vi "Reset VFD.vi"(6 "Direction":T1=2 items=["Reverse"=0, "Forward"=2], 8 "error In":errorcluster) -> (0 "error out":errorcluster)   [LabVIEW 2026, in "VFD Library.lvlib"]
uses:
  VFD Library.lvlib
  Action/Direction Selection.ctl
  Private/State Selection FGV.ctl
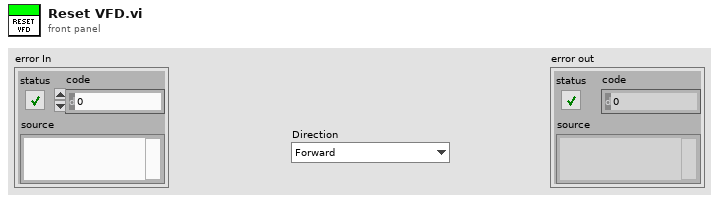
[diagram p1: front panel]
types:
  T1 = typedef "VFD Library.lvlib/Direction Selection.ctl" = u16
  T2 = typedef "State Selection FGV.ctl" = enum16{"Initilize", "Write Reg", "Write Multiple Reg", "Read Reg", "Write Coil", "Read Coil", "Reset", "Close"}
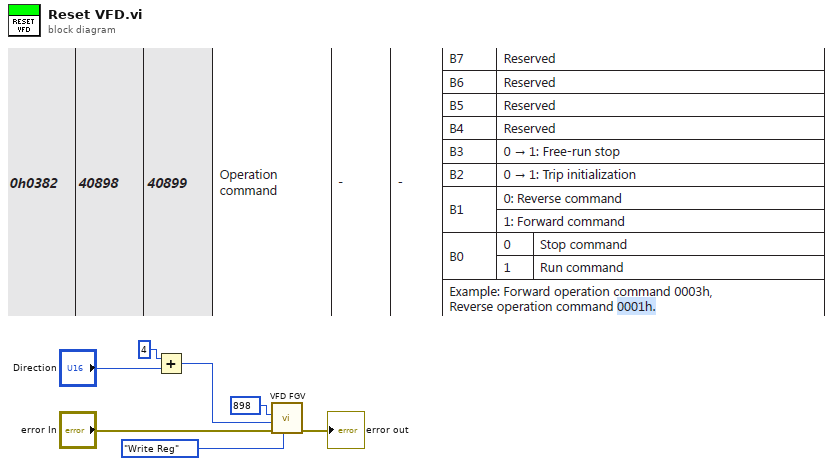
[diagram p0: block diagram]
diagram:
  n1 = Add(x=u16 4 ("value"), y="Direction") -> (x+y=w2:T1)
  n2 = call "VFD FGV.vi"("State"=State_Selection_FGV."Write Reg", "error In"="error In", "value"=w2, "address"=u16 898) -> ("error out"=→"error out":errorcluster)  [unwired: 5 in, 2 out]
